vi "Configure Sweep (Transient).vi"(0 "VISA resource name":refnum<visa-resource-name>, 1 "Narrow Span (100E-3 s)":dbl=0.1 format="%^#_9g", 2 "Narrow Time Offset (0 s)":dbl format="%^#_9g", 5 "Wide Span (100E-3 s)":dbl=0.1 format="%^#_9g", 7 "Wide Reference Position (1: Center)":u16(ring)=1 items=["Left", "Center", "Right"], 9 "Wide Time Offset (0 s)":dbl format="%^#_9g", 11 "error in (no error)":errorcluster, 12 "Narrow Reference Position (1: Center)":u16(ring)=1 items=["Left", "Center", "Right"]) -> (4 "VISA resource name out":refnum<visa-resource-name>, 15 "error out":errorcluster)   [LabVIEW 2011, in "Agilent E5052X.lvlib"]
doc: "Sets the range in which measurements will be taken for the Transient measurement.\n\n<b>Note:</b>\n\n1) \"Configure Measurement Characteristics(Transient)\" VI must be run before this VI."
uses:
  Agilent E5052X.lvlib
panel:
  # "Wideband Trace Settings"
  # "Narrowband Trace Settings"
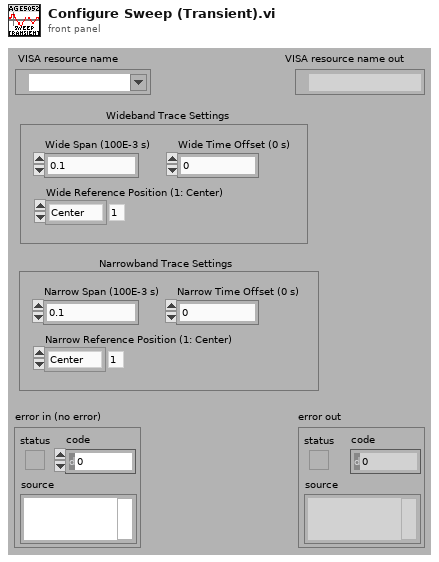
[diagram p1: front panel]
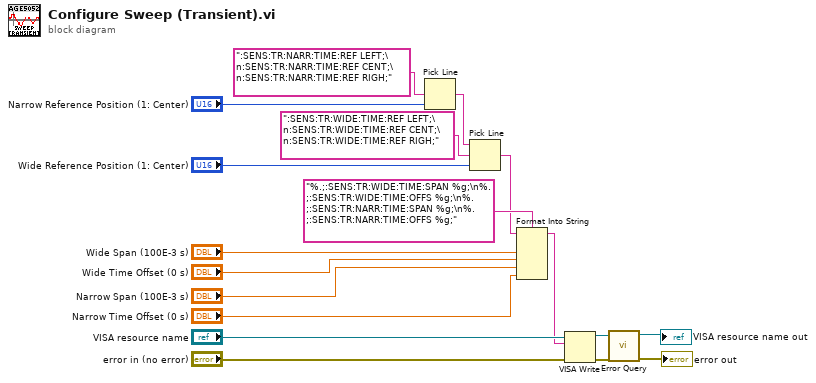
[diagram p0: block diagram]
diagram:
  n1 = Pick Line(multi-line string=":SENS:TR:NARR:TIME:REF LEFT;\n:SENS:TR:NARR:TIME:REF CENT;\n:SENS:TR:NARR:TIME:REF RIGH;", line index="Narrow Reference Position (1: Center)") -> (output string=w3:string)  [unwired: 1 in]
  n2 = Pick Line(string ("")=w3, multi-line string=":SENS:TR:WIDE:TIME:REF LEFT;\n:SENS:TR:WIDE:TIME:REF CENT;\n:SENS:TR:WIDE:TIME:REF RIGH;", line index="Wide Reference Position (1: Center)") -> (output string=w2:string)
  n3 = Format Into String(format string="%.;:SENS:TR:WIDE:TIME:SPAN %g;\n%.;:SENS:TR:WIDE:TIME:OFFS %g;\n%.;:SENS:TR:NARR:TIME:SPAN %g;\n%.;:SENS:TR:NARR:TIME:OFFS %g;", initial string=w2, "Wide Span (100E-3 s)", "Wide Time Offset (0 s)", "Narrow Span (100E-3 s)", "Narrow Time Offset (0 s)") -> (resulting string=w1:string)  [unwired: 1 in, 1 out]
  n4 = VISA Write(VISA resource name="VISA resource name", write buffer=w1, error in (no error)="error in (no error)") -> (VISA resource name out=w11:refnum<visa-resource-name>, error out=w10:errorcluster)  [unwired: 1 out]
  n5 = call "Error Query.vi"("error in (no error)"=w10, "VISA resource name"=w11) -> ("error out"=→"error out":errorcluster, "VISA resource name out"=→"VISA resource name out":refnum<visa-resource-name>)  [unwired: 6 in, 2 out]
